vi "CRYAna Hetero.vi"(0 "Calibration Response Cluster":T1={"Calibration"={"Calibration Step Name"="", "Device"="", "Correction Curve Name"="", "Equalization Curve Name"="", "Sensitivity Curve Name"="", "Corr Folder and File"="", "EQ Folder and File"="", "Sens Folder and File"="", "Corr Step size"=0, "EQ Step size"=0, "Input"=FALSE, "Last Cal Date (sec)"=timestamp(0 s since 1904-01-01), "Cha Name"="", "Corr Curve Found"=FALSE, "EQ Curve Found"=FALSE, "Sens Curve Found"=FALSE, "Signal Type"="", "Calibrated Device"="", "Hz"=0}, "Corr Curve"={"Name"="", "Curve"=[], "X data"=1, "Y data"=1, "Z data"=1, "X axis"=0, "Y axis"=1, "Z axis"=1, "X unit"="Hz", "Y unit"="", "Z unit"="deg.", "X dB ref"=1.0, "Y dB ref"=1.0, "Z dB ref"=1.0, "single val"=FALSE, "protected"=FALSE, "display X"=TRUE, "display Y"=TRUE, "display Z"=TRUE, "Test Info"="", "Step No."=0, "Plot Settings"={"Color"=0, "Interpolation"=0, "Point Style"=0, "Line Style"=0, "Point Color"=0, "Line Width"=0, "Bar Plot Style"=0, "Fill To"=0}, "AutoProtect"=FALSE}, "EQ Curve"={"Name"="", "Curve"=[], "X data"=1, "Y data"=1, "Z data"=1, "X axis"=0, "Y axis"=1, "Z axis"=1, "X unit"="Hz", "Y unit"="", "Z unit"="deg.", "X dB ref"=1.0, "Y dB ref"=1.0, "Z dB ref"=1.0, "single val"=FALSE, "protected"=FALSE, "display X"=TRUE, "display Y"=TRUE, "display Z"=TRUE, "Test Info"="", "Step No."=0, "Plot Settings"={"Color"=0, "Interpolation"=0, "Point Style"=0, "Line Style"=0, "Point Color"=0, "Line Width"=0, "Bar Plot Style"=0, "Fill To"=0}, "AutoProtect"=FALSE}, "Sens Curve"={"Name"="", "Curve"=[], "X data"=1, "Y data"=1, "Z data"=1, "X axis"=0, "Y axis"=1, "Z axis"=1, "X unit"="Hz", "Y unit"="", "Z unit"="deg.", "X dB ref"=1.0, "Y dB ref"=1.0, "Z dB ref"=1.0, "single val"=FALSE, "protected"=FALSE, "display X"=TRUE, "display Y"=TRUE, "display Z"=TRUE, "Test Info"="", "Step No."=0, "Plot Settings"={"Color"=0, "Interpolation"=0, "Point Style"=0, "Line Style"=0, "Point Color"=0, "Line Width"=0, "Bar Plot Style"=0, "Fill To"=0}, "AutoProtect"=FALSE}} {"Sens Curve"."Z data" items=["dB", "Lin"]; "Sens Curve"."X data" items=["dB", "Lin"]; "Sens Curve"."Y data" items=["dB", "Lin"]; "Sens Curve"."Z dB ref" format="%.1f"; "Sens Curve"."Z axis" items=["Log", "Lin"]; "Sens Curve"."X dB ref" format="%.1f"; "Sens Curve"."X axis" items=["Log", "Lin"]; "Sens Curve"."Y axis" items=["Log", "Lin"]; "Sens Curve"."Y dB ref" format="%.1f"; "Sens Curve"."Curve"."z" format="%.2f"; "Sens Curve"."Curve"."y" format="%.2f"; "Sens Curve"."Curve"."x" format="%.2f"; "EQ Curve"."Z data" items=["dB", "Lin"]; "EQ Curve"."X data" items=["dB", "Lin"]; "EQ Curve"."Y data" items=["dB", "Lin"]; "EQ Curve"."Z dB ref" format="%.1f"; "EQ Curve"."Z axis" items=["Log", "Lin"]; "EQ Curve"."X dB ref" format="%.1f"; "EQ Curve"."X axis" items=["Log", "Lin"]; "EQ Curve"."Y axis" items=["Log", "Lin"]; "EQ Curve"."Y dB ref" format="%.1f"; "EQ Curve"."Curve"."z" format="%.2f"; "EQ Curve"."Curve"."y" format="%.2f"; "EQ Curve"."Curve"."x" format="%.2f"; "Corr Curve"."Z data" items=["dB", "Lin"]; "Corr Curve"."X data" items=["dB", "Lin"]; "Corr Curve"."Y data" items=["dB", "Lin"]; "Corr Curve"."Z dB ref" format="%.1f"; "Corr Curve"."Z axis" items=["Log", "Lin"]; "Corr Curve"."X dB ref" format="%.1f"; "Corr Curve"."X axis" items=["Log", "Lin"]; "Corr Curve"."Y axis" items=["Log", "Lin"]; "Corr Curve"."Y dB ref" format="%.1f"; "Corr Curve"."Curve"."z" format="%.2f"; "Corr Curve"."Curve"."y" format="%.2f"; "Corr Curve"."Curve"."x" format="%.2f"; "Calibration"."EQ Step size" items=["R10", "R20", "R40", "R80", "User"]; "Calibration"."Corr Step size" items=["R10", "R20", "R40", "R80", "User"]}, 4 "Distortion Infor":T6, 5 "Calibration Stimulus Cluster":T1={"Calibration"={"Calibration Step Name"="", "Device"="", "Correction Curve Name"="", "Equalization Curve Name"="", "Sensitivity Curve Name"="", "Corr Folder and File"="", "EQ Folder and File"="", "Sens Folder and File"="", "Corr Step size"=0, "EQ Step size"=0, "Input"=FALSE, "Last Cal Date (sec)"=timestamp(0 s since 1904-01-01), "Cha Name"="", "Corr Curve Found"=FALSE, "EQ Curve Found"=FALSE, "Sens Curve Found"=FALSE, "Signal Type"="", "Calibrated Device"="", "Hz"=0}, "Corr Curve"={"Name"="", "Curve"=[], "X data"=1, "Y data"=1, "Z data"=1, "X axis"=0, "Y axis"=1, "Z axis"=1, "X unit"="Hz", "Y unit"="", "Z unit"="deg.", "X dB ref"=1.0, "Y dB ref"=1.0, "Z dB ref"=1.0, "single val"=FALSE, "protected"=FALSE, "display X"=TRUE, "display Y"=TRUE, "display Z"=TRUE, "Test Info"="", "Step No."=0, "Plot Settings"={"Color"=0, "Interpolation"=0, "Point Style"=0, "Line Style"=0, "Point Color"=0, "Line Width"=0, "Bar Plot Style"=0, "Fill To"=0}, "AutoProtect"=FALSE}, "EQ Curve"={"Name"="", "Curve"=[], "X data"=1, "Y data"=1, "Z data"=1, "X axis"=0, "Y axis"=1, "Z axis"=1, "X unit"="Hz", "Y unit"="", "Z unit"="deg.", "X dB ref"=1.0, "Y dB ref"=1.0, "Z dB ref"=1.0, "single val"=FALSE, "protected"=FALSE, "display X"=TRUE, "display Y"=TRUE, "display Z"=TRUE, "Test Info"="", "Step No."=0, "Plot Settings"={"Color"=0, "Interpolation"=0, "Point Style"=0, "Line Style"=0, "Point Color"=0, "Line Width"=0, "Bar Plot Style"=0, "Fill To"=0}, "AutoProtect"=FALSE}, "Sens Curve"={"Name"="", "Curve"=[], "X data"=1, "Y data"=1, "Z data"=1, "X axis"=0, "Y axis"=1, "Z axis"=1, "X unit"="Hz", "Y unit"="", "Z unit"="deg.", "X dB ref"=1.0, "Y dB ref"=1.0, "Z dB ref"=1.0, "single val"=FALSE, "protected"=FALSE, "display X"=TRUE, "display Y"=TRUE, "display Z"=TRUE, "Test Info"="", "Step No."=0, "Plot Settings"={"Color"=0, "Interpolation"=0, "Point Style"=0, "Line Style"=0, "Point Color"=0, "Line Width"=0, "Bar Plot Style"=0, "Fill To"=0}, "AutoProtect"=FALSE}} {"Sens Curve"."Z data" items=["dB", "Lin"]; "Sens Curve"."X data" items=["dB", "Lin"]; "Sens Curve"."Y data" items=["dB", "Lin"]; "Sens Curve"."Z dB ref" format="%.1f"; "Sens Curve"."Z axis" items=["Log", "Lin"]; "Sens Curve"."X dB ref" format="%.1f"; "Sens Curve"."X axis" items=["Log", "Lin"]; "Sens Curve"."Y axis" items=["Log", "Lin"]; "Sens Curve"."Y dB ref" format="%.1f"; "Sens Curve"."Curve"."z" format="%.2f"; "Sens Curve"."Curve"."y" format="%.2f"; "Sens Curve"."Curve"."x" format="%.2f"; "EQ Curve"."Z data" items=["dB", "Lin"]; "EQ Curve"."X data" items=["dB", "Lin"]; "EQ Curve"."Y data" items=["dB", "Lin"]; "EQ Curve"."Z dB ref" format="%.1f"; "EQ Curve"."Z axis" items=["Log", "Lin"]; "EQ Curve"."X dB ref" format="%.1f"; "EQ Curve"."X axis" items=["Log", "Lin"]; "EQ Curve"."Y axis" items=["Log", "Lin"]; "EQ Curve"."Y dB ref" format="%.1f"; "EQ Curve"."Curve"."z" format="%.2f"; "EQ Curve"."Curve"."y" format="%.2f"; "EQ Curve"."Curve"."x" format="%.2f"; "Corr Curve"."Z data" items=["dB", "Lin"]; "Corr Curve"."X data" items=["dB", "Lin"]; "Corr Curve"."Y data" items=["dB", "Lin"]; "Corr Curve"."Z dB ref" format="%.1f"; "Corr Curve"."Z axis" items=["Log", "Lin"]; "Corr Curve"."X dB ref" format="%.1f"; "Corr Curve"."X axis" items=["Log", "Lin"]; "Corr Curve"."Y axis" items=["Log", "Lin"]; "Corr Curve"."Y dB ref" format="%.1f"; "Corr Curve"."Curve"."z" format="%.2f"; "Corr Curve"."Curve"."y" format="%.2f"; "Corr Curve"."Curve"."x" format="%.2f"; "Calibration"."EQ Step size" items=["R10", "R20", "R40", "R80", "User"]; "Calibration"."Corr Step size" items=["R10", "R20", "R40", "R80", "User"]}, 6 "Stimulus Infor":T4, 8 "Time Infor":cluster{"window":u16, "discard cycles":dbl}={"window"=0, "discard cycles"=3.0} {"discard cycles" min=1.0}, 9 "Wave Infor":T5 {"Sens In" format="%.2f"; "Response(Abs/Rel)" items=["Absolute", "Relative"]}, 10 "Response":dbl[](array[numeric]), 11 "Algorithm":u16) -> (1 "Freq resp curves clipped":cluster{cluster{"x":dbl, "y":dbl, "z":dbl}[]}[](array[cluster]) {"?"."y" format="%#_6p"}, 3 "Corrected Response Out":dbl[](array[numeric]))   [LabVIEW 2013]
uses:
  Typedef Control/CRYCalibration 2DCluster.ctl
  Typedef Control/CRYCalibration Cluster.ctl
  Typedef Control/CRYData Cluster.ctl
  <vilib>/Analysis/0measdsp.llb/Scaled Time Domain Window (DBL).vi
  <vilib>/Analysis/baseanly.llb/Mean (CDB).vi
  <vilib>/Analysis/NI_AALBase.lvlib
  <vilib>/Analysis/NI_AALPro.lvlib
panel:
  out "Waveform Graph":dbl[](graph)
  out "XY Graph":cluster{cluster{"Fi":dbl, dbl}[]}[](graph)
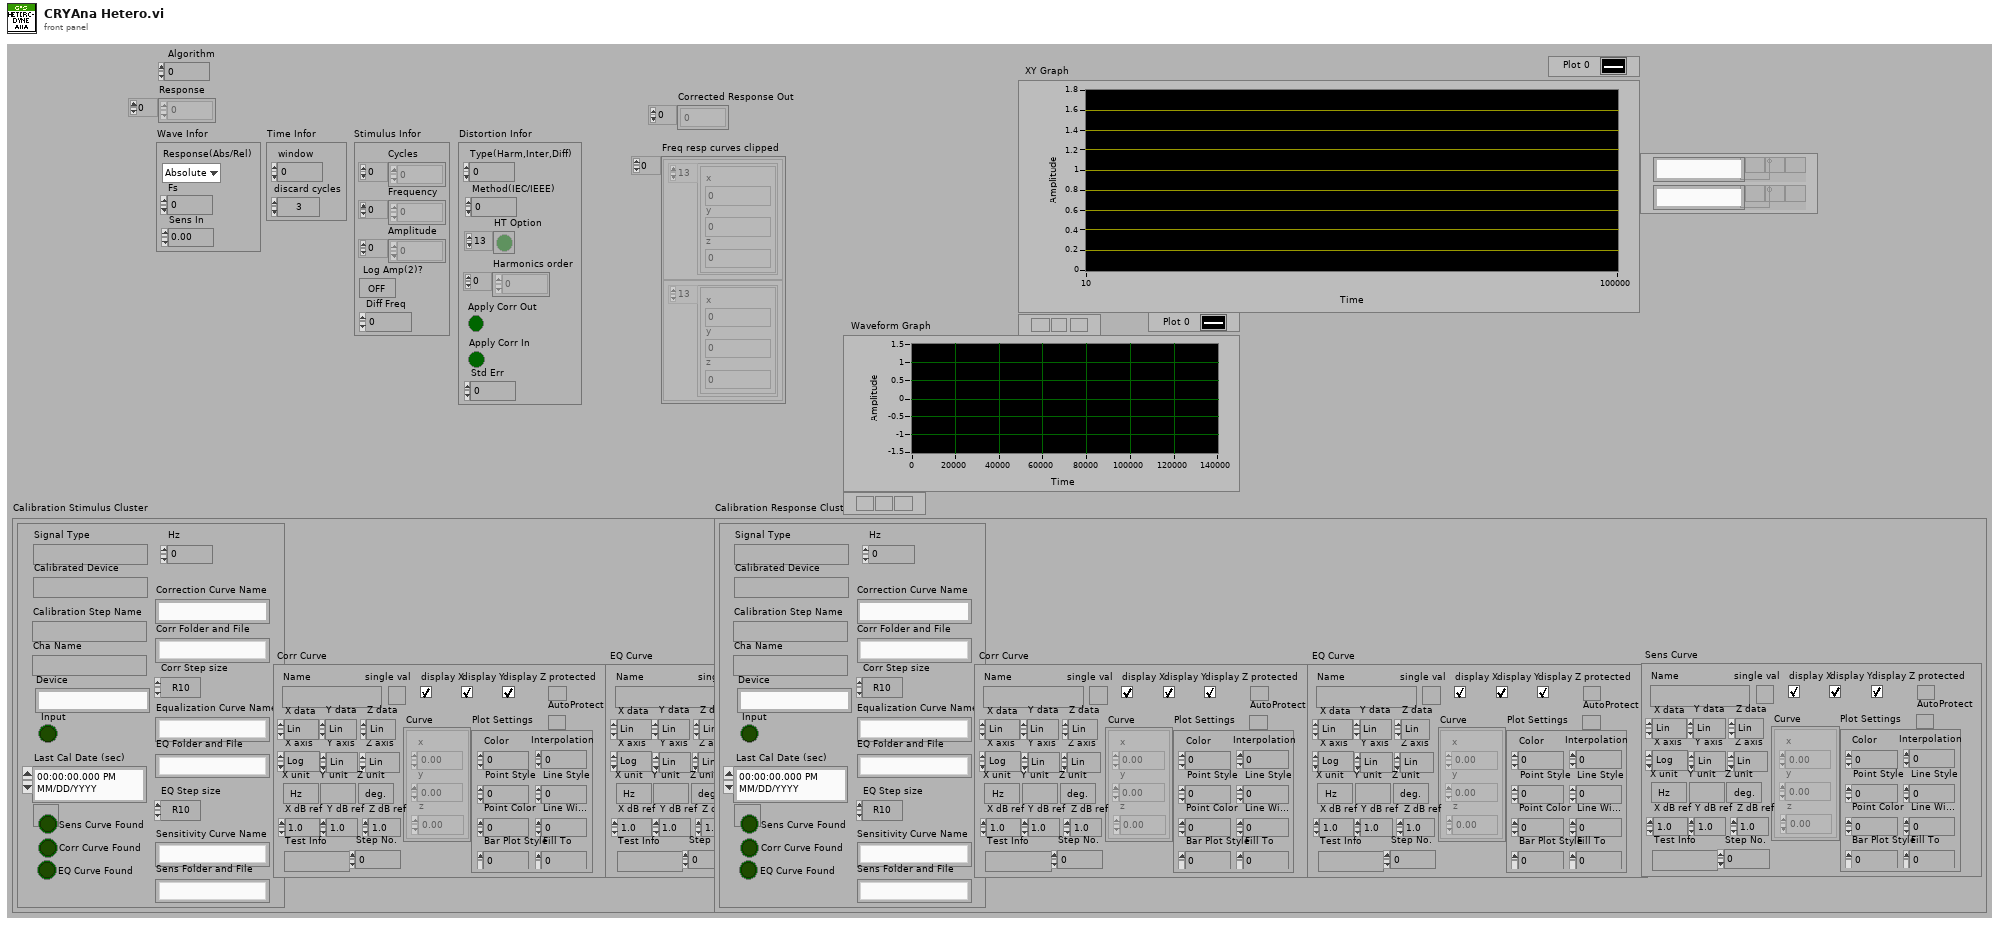
[diagram p1: front panel]
types:
  T1 = typedef "CRYCalibration 2DCluster.ctl" = cluster{"Calibration":T2, "Corr Curve":T3, "EQ Curve":T3, "Sens Curve":T3}
  T2 = typedef "CRYCalibration Cluster.ctl" = cluster{"Calibration Step Name":string, "Device":string, "Correction Curve Name":string, "Equalization Curve Name":string, "Sensitivity Curve Name":string, "Corr Folder and File":string, "EQ Folder and File":string, "Sens Folder and File":string, "Corr Step size":u16, "EQ Step size":u16, "Input":bool, "Last Cal Date (sec)":timestamp, "Cha Name":string, "Corr Curve Found":bool, "EQ Curve Found":bool, "Sens Curve Found":bool, "Signal Type":string, "Calibrated Device":string, "Hz":u32}
  T3 = typedef "CRYData Cluster.ctl" = cluster{"Name":string, "Curve":cluster{"x":dbl, "y":dbl, "z":dbl}[], "X data":u16, "Y data":u16, "Z data":u16, "X axis":u16, "Y axis":u16, "Z axis":u16, "X unit":string, "Y unit":string, "Z unit":string, "X dB ref":dbl, "Y dB ref":dbl, "Z dB ref":dbl, "single val":bool, "protected":bool, "display X":bool, "display Y":bool, "display Z":bool, "Test Info":string, "Step No.":i32, "Plot Settings":cluster{"Color":u32, "Interpolation":u8, "Point Style":u8, "Line Style":u8, "Point Color":u32, "Line Width":u8, "Bar Plot Style":u8, "Fill To":i16}, "AutoProtect":bool}
  T4 = cluster{"Cycles":dbl[], "Frequency":dbl[], "Amplitude":dbl[], " Log Amp(2)?":bool, "Diff Freq":dbl}
  T5 = cluster{"Response(Abs/Rel)":u16, "Fs":dbl, "Sens In":dbl}
  T6 = cluster{"Type(Harm,Inter,Diff)":u16, "Method(IEC/IEEE)":u16, "HT Option":bool[], "Harmonics order":dbl[], "Apply Corr Out":bool, "Apply Corr In":bool, "Std Err":dbl}
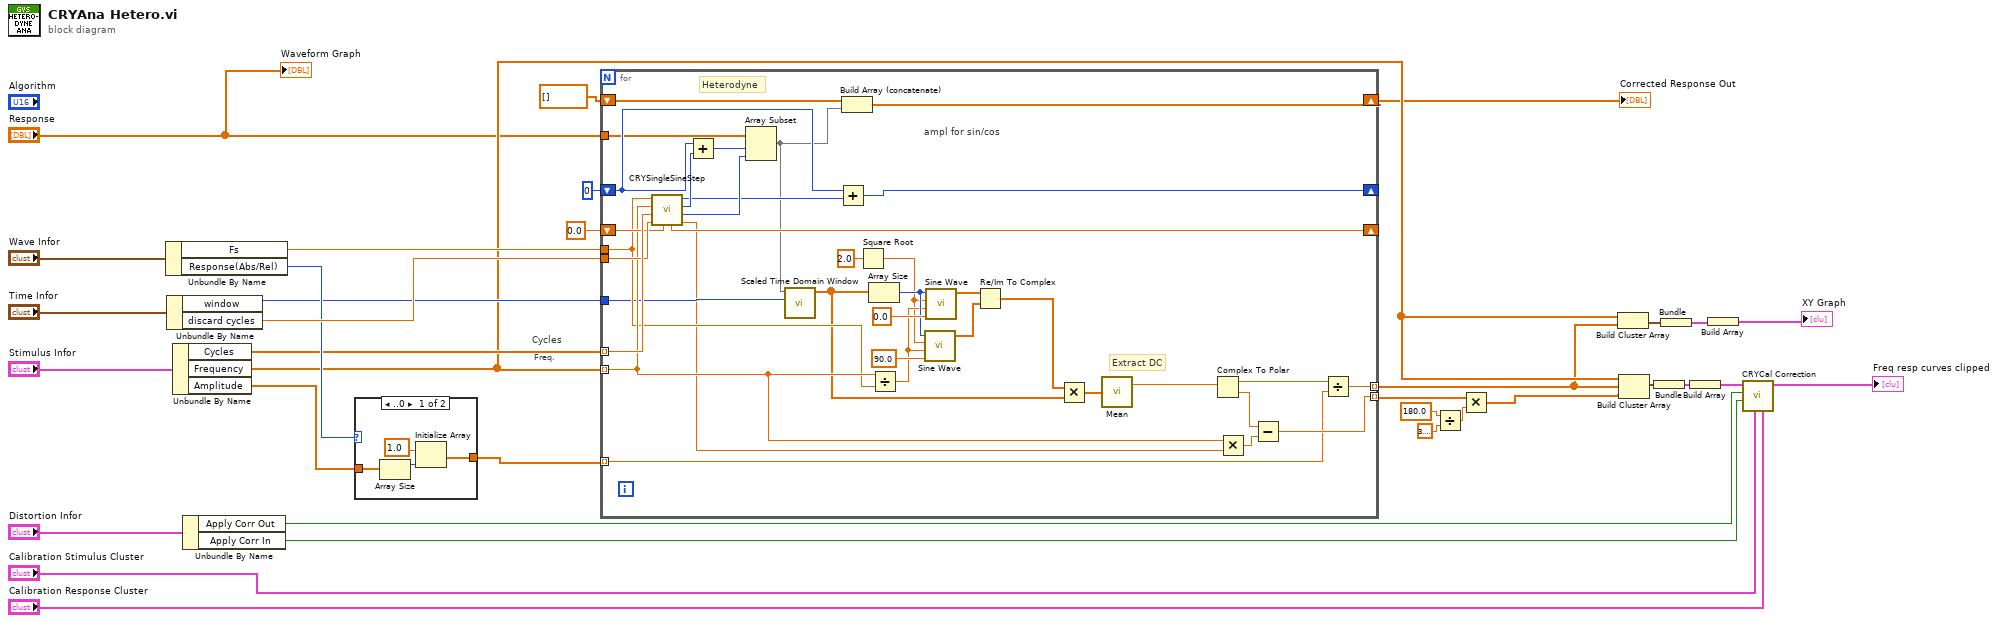
[diagram p0: block diagram]
diagram:
  # "Cycles"
  # "Freq."
  n1 = Unbundle By Name("Wave Infor") -> ("Fs"=w21:dbl, "Response(Abs/Rel)"=w27:u16)
  n2 = Unbundle By Name("Time Infor") -> ("window"=w22:u16, "discard cycles"=w30:dbl)
  n3 = Unbundle By Name("Stimulus Infor") -> ("Cycles"=w25:dbl[], "Frequency"=w5:dbl[], "Amplitude"=w24:dbl[])
  n4 = Unbundle By Name("Distortion Infor") -> ("Apply Corr Out"=w18:bool, "Apply Corr In"=w17:bool)
  n5 = case shown="..0" w27 {
    tunnel: [w35 w39] -> w23
    tunnel: w24 -> [w38 w39]
    frame ..0 {
      n6 = Array Size(array=w38) -> (size(s)=w37:i32)
      n7 = Initialize Array(1.0 ("Level left"), w37) -> (w35:dbl[])
    }
    frame 1.. {
    }
  }
  n8 = for {
    tunnel: w21 -> [w65]
    shift-right: [w74] -> _
    shift-left: 0 -> [w73]
    tunnel: "Response" -> [w66]
    shift-right: [w75] -> w3
    shift-left: dbl[] [] -> [w69]
    tunnel: w25 -> [w72] mode=indexing
    tunnel: w5 -> [w67] mode=indexing
    tunnel: w23 -> [w43] mode=indexing
    tunnel: w30 -> [w71]
    shift-right: [w68] -> _
    shift-left: 0.0 -> [w70]
    tunnel: w22 -> [w57]
    tunnel: [w55] -> w2 mode=indexing
    tunnel: [w50] -> w6 mode=indexing
    # "Heterodyne"
    # "ampl for sin/cos"
    # "Extract DC"
    n9 = call "CRYSingleSineStep.vi"("Fs"=w65, "Freq"=w67, "Cycles per freq"=w72, "Cycles discarded"=w71, "StartPhase"=w70) -> ("StopPhase"=w68:dbl, "TotalSamples"=w51:i32, "DiscardSamples"=w58:i32, "ExtractSamples"=w52:i32, "TimeCorrection"=w48:dbl)  [unwired: 1 out]
    n10 = Add(x=w73, y=w58) -> (x+y=w53:i32)
    n11 = Array Subset(array=w66, index=w53, length=w52) -> (w40:dbl[])
    n12 = call-poly <vilib>:"Scaled Time Domain Window.vi"("window"=w57, "X"=w40) -> ("Windowed X"=w44:dbl[])  [unwired: 7 in, 2 out]
    n13 = Add(x=w73, y=w51) -> (x+y=w74:i32)
    n14 = Build Array (concatenate)(w69, w40) -> (w75:dbl[])
    n15 = Square Root(x=2.0) -> (sqrt(x)=w56:dbl)
    n16 = Array Size(array=w44) -> (size(s)=w60:i32)
    n17 = Divide(x=w67, y=w65) -> (x/y=w59:dbl)
    n18 = call <vilib>:"Sine Wave.vi"("samples"=w60, "amplitude"=w56, "frequency"=w59, "phase in"=90.0) -> ("sine wave"=w49:dbl[])  [unwired: 1 in, 2 out]
    n19 = call <vilib>:"Sine Wave.vi"("samples"=w60, "amplitude"=w56, "frequency"=w59, "phase in"=0.0) -> ("sine wave"=w41:dbl[])  [unwired: 1 in, 2 out]
    n20 = Re/Im To Complex(1:w49, 2:w41) -> (0:w47:cdb[])
    n21 = Multiply(x=w47, y=w44) -> (x*y=w45:cdb[])
    n22 = call-poly <vilib>:"Mean.vi"("X"=w45) -> ("mean"=w46:cdb)  [unwired: 1 out]
    n23 = Complex To Polar(r * e^(i*theta)=w46) -> (r=w54:dbl, theta=w42:dbl)
    n24 = Multiply(x=w67, y=w48) -> (x*y=w62:dbl)
    n25 = Subtract(x=w42, y=w62) -> (x-y=w50:dbl)
    n26 = Divide(x=w54, y=w43) -> (x/y=w55:dbl)
  }
  "Corrected Response Out" <- w3
  n27 = Divide(x=180.0, y=3.141592653589793) -> (x/y=w16:dbl)
  n28 = Multiply(x=w6, y=w16) -> (x*y=w4:dbl[])
  n29 = Build Cluster Array(w5, w2) -> (w9:cluster{"Fi":dbl, dbl}[])
  n30 = Build Cluster Array(w5, w2, w4) -> (w13:cluster{"Fi":dbl, dbl, dbl}[])
  n31 = Bundle(w13) -> (w12:cluster{cluster{"Fi":dbl, dbl, dbl}[]})  [unwired: 1 in]
  n32 = Bundle(w9) -> (w8:cluster{cluster{"Fi":dbl, dbl}[]})  [unwired: 1 in]
  n33 = Build Array(w12) -> (w10:cluster{cluster{"Fi":dbl, dbl, dbl}[]}[])
  n34 = Build Array(w8) -> (→"XY Graph":cluster{cluster{"Fi":dbl, dbl}[]}[])
  n35 = call "CRYCal Correction.vi"("Calibration Response Cluster"="Calibration Response Cluster", "Calibration Stimulus Cluster"="Calibration Stimulus Cluster", "Apply Corr In"=w17, "Apply Corr Out"=w18, "Frequency curve in"=w10) -> ("Frequency curve out"=→"Freq resp curves clipped":cluster{cluster{"x":dbl, "y":dbl, "z":dbl}[]}[])  [unwired: 6 in]
  "Waveform Graph" <- "Response"
